vi "Destroy MeasData Q.vi"(8 "error in (no error)":errorcluster, 10 "wait for activity?":bool) -> (0 "error out":errorcluster, 3 "final data":T1)   [LabVIEW 2020]
doc: "Developed by Kevin Thompson\nThompson Engineering, LLC\nkevin@thompsonengineering.net"
uses:
  GBL DataQ Ref.vi
  TD MeasData--cluster.ctl
  TD MeasData QRef.ctl
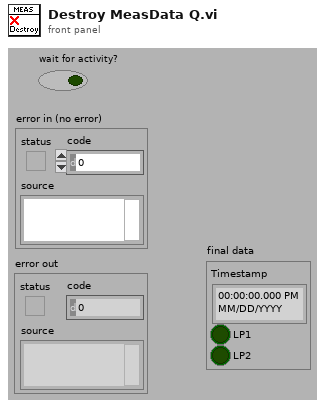
[diagram p1: front panel]
types:
  T1 = typedef "TD MeasData--cluster.ctl" = cluster{"Timestamp":timestamp, "LP1":bool, "LP2":bool}
  T2 = typedef "TD MeasData QRef.ctl" = refnum<queue>
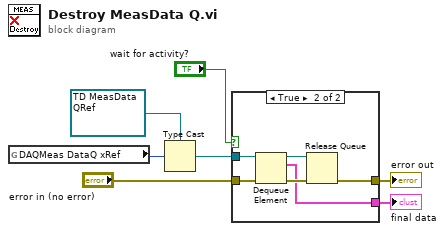
[diagram p0: block diagram]
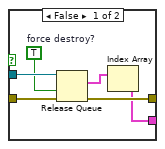
[diagram p2: hidden frame]
diagram:
  n1 = global read "GBL DataQ Ref.vi" "DAQMeas DataQ xRef"() -> (w2:u32)
  n2 = Type Cast(type=T2 refnum ("MeasDataQRef"), x=w2) -> (*(type *) &x=w4:T2)
  n3 = case shown="True" "wait for activity?" {
    tunnel: "error in (no error)" -> [w11 w19]
    tunnel: w4 -> [w10 w18]
    tunnel: [w13 w15] -> w6
    tunnel: [w8 w14] -> w3
    frame False {
      w9 = TRUE  # force destroy?
      n4 = Release Queue(queue=w10, force destroy? (F)=w9, error in (no error)=w11) -> (remaining elements=w12:T1[], error out=w13:errorcluster)  [unwired: 1 out]
      n5 = Index Array(array=w12) -> (element=w8:T1)  [unwired: 1 in]
    }
    frame True {
      n6 = Dequeue Element(queue=w18, error in (no error)=w19) -> (queue out=w16:T2, element=w14:T1, error out=w17:errorcluster)  [unwired: 1 in, 1 out]
      n7 = Release Queue(queue=w16, error in (no error)=w17) -> (error out=w15:errorcluster)  [unwired: 1 in, 2 out]
    }
  }
  "final data" <- w3
  "error out" <- w6
